vi "read coils.vi"(8 "error in (no error)":errorcluster, 10 "quantity":u16, 11 "starting address":u16) -> (0 "error out":errorcluster, 3 "Coils":bool[](array[boolean]))   [LabVIEW 2016, in "环境动力监测库.lvlib" / "浮标电源管理.lvlib"]
uses:
  <vilib>/Plasmionique/MB Master/MB Master.lvlib
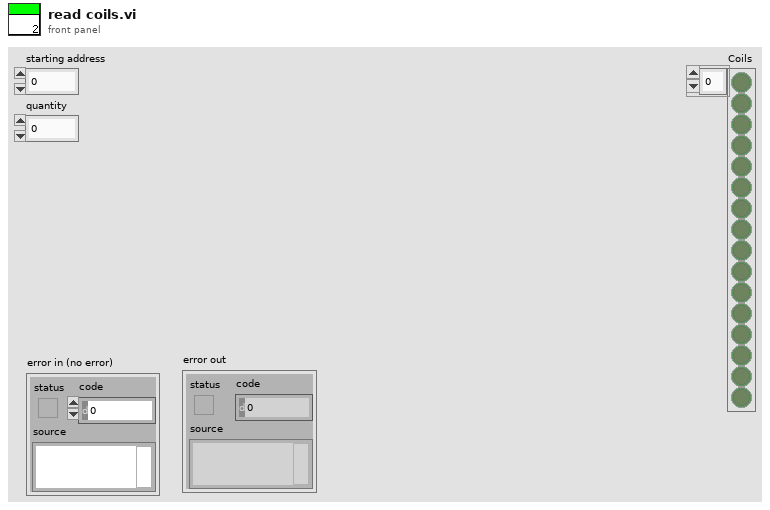
[diagram p1: front panel]
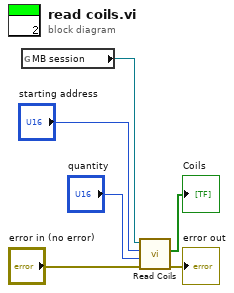
[diagram p0: block diagram]
diagram:
  n1 = global read "通讯全局变量.vi" "MB session"() -> (w6:refnum<class "MB_Master.lvclass">)
  n2 = call <vilib>:"Read Coils.vi"("error in (no error)"="error in (no error)", "quantity"="quantity", "starting address"="starting address", "MB session in"=w6) -> ("error out"=→"error out":errorcluster, "Coils"=→"Coils":bool[])  [unwired: 5 in, 1 out]
